vi "Lab Panel V4.85.vi"() -> ()   [LabVIEW 2013] (continued)
                    n1929 = Unbundle By Name(w3325) -> ("1  (A) cal"=w3318:dbl, "1 (V) cal"=w3317:dbl, "1 (PF) cal"=w3316:dbl, "2 (A) cal"=w3315:dbl, "2 (V) cal"=w3314:dbl, "2 (PF) cal"=w3313:dbl)  [unwired: 4 out]
                    n1930 = Multiply(x=w3324, y=w3318) -> (x*y=w3311:dbl)
                    n1931 = Multiply(x=w3323, y=w3317) -> (x*y=w3310:dbl)
                    n1932 = Multiply(x=w3322, y=w3316) -> (x*y=w3309:dbl)
                    n1933 = Multiply(x=w3321, y=w3315) -> (x*y=w3307:dbl)
                    n1934 = Multiply(x=w3320, y=w3314) -> (x*y=w3306:dbl)
                    n1935 = Multiply(x=w3319, y=w3313) -> (x*y=w3305:dbl)
                    n1936 = local read "SIG LAB04-1"() -> (w3312:T2)
                    n1937 = local read "SIG LAB04-2"() -> (w3308:T2)
                    n1938 = Bundle By Name(cluster=w3312, "AMPS"=w3311, "VOLTS"=w3310, "PF"=w3309) -> (w3301:T2)
                    n1939 = Bundle By Name(cluster=w3308, "AMPS"=w3307, "VOLTS"=w3306, "PF"=w3305) -> (w3300:T2)
                    n1940 = global write "Global display 1.vi" "SIG LAB04-2"(w3300) -> ()
                    n1941 = global write "Global display 1.vi" "SIG LAB04-1"(w3301) -> ()
                    n1942 = local write "SIG LAB04-2"(w3300) -> ()
                    n1943 = local write "SIG LAB04-1"(w3301) -> ()
                  }
                  frame #5 {
                    n1944 = Unbundle By Name(w3333) -> ("LAB05-1 (A)"=w3352:dbl, "LAB05-1 (V)"=w3332:dbl, "LAB05-1 (PF)"=w3351:dbl, "LAB05-2 (A)"=w3350:dbl, "LAB05-2 (V)"=w3349:dbl, "LAB05-2 (PF)"=w3348:dbl)
                    n1945 = case shown="False" w3331 {
                      tunnel: [w3354 w3355] -> w3353
                      tunnel: w3330 -> [_ w3355]
                      frame False {
                        n1946 = local read "CAL LAB05"() -> (w3354:T12)
                      }
                      frame True {
                      }
                    }
                    n1947 = Unbundle By Name(w3353) -> ("1  (A) cal"=w3347:dbl, "1 (V) cal"=w3346:dbl, "1 (PF) cal"=w3345:dbl, "2 (A) cal"=w3344:dbl, "2 (V) cal"=w3343:dbl, "2 (PF) cal"=w3342:dbl)  [unwired: 4 out]
                    n1948 = Multiply(x=w3352, y=w3347) -> (x*y=w3340:dbl)
                    n1949 = Multiply(x=w3332, y=w3346) -> (x*y=w3339:dbl)
                    n1950 = Multiply(x=w3351, y=w3345) -> (x*y=w3338:dbl)
                    n1951 = Multiply(x=w3350, y=w3344) -> (x*y=w3336:dbl)
                    n1952 = Multiply(x=w3349, y=w3343) -> (x*y=w3335:dbl)
                    n1953 = Multiply(x=w3348, y=w3342) -> (x*y=w3334:dbl)
                    n1954 = local read "SIG LAB05-1"() -> (w3341:T2)
                    n1955 = local read "SIG LAB05-2"() -> (w3337:T2)
                    n1956 = Bundle By Name(cluster=w3341, "AMPS"=w3340, "VOLTS"=w3339, "PF"=w3338) -> (w3329:T2)
                    n1957 = Bundle By Name(cluster=w3337, "AMPS"=w3336, "VOLTS"=w3335, "PF"=w3334) -> (w3328:T2)
                    n1958 = global write "Global display 1.vi" "SIG LAB05-1"(w3329) -> ()
                    n1959 = global write "Global display 1.vi" "SIG LAB05-2"(w3328) -> ()
                    n1960 = local write "SIG LAB05-2"(w3328) -> ()
                    n1961 = local write "SIG LAB05-1"(w3329) -> ()
                  }
                }
              }
            }
          }
          frame #12 {
            # "save test data to file"
            n1962 = Get Date/Time In Seconds() -> (seconds since 1Jan1904=w3356:timestamp)
            "File Time Stamp" <- w3356
            n1963 = local read "on loops"() -> (w3375:dbl)
            n1964 = local read "jig cycle"() -> (w3372:dbl)
            n1965 = Format Date/Time String(time format string (%c)="%H:%M%:%S", seconds (now)=w3356) -> (date/time string=w3360:string)  [unwired: 1 in]
            n1966 = Add(x=w3375, y=2) -> (x+y=w3373:dbl)
            n1967 = Build Array(w3360) -> (w3359:string[])
            n1968 = Equal?(x=w3372, y=1) -> (x = y?=w3358:bool)
            n1969 = Equal?(x=w3372, y=w3373) -> (x = y?=w3357:bool)
            n1970 = stacked-sequence {
              tunnel: w3371 -> [w3381 _ _ _ _ _ _ _ _ _]
              tunnel: w3370 -> [_ w3457 _ _ _ _ _ _ _ _]
              tunnel: w3369 -> [_ _ w3537 _ _ _ _ _ _ _]
              tunnel: w3368 -> [_ _ _ w3617 _ _ _ _ _ _]
              tunnel: w3367 -> [_ _ _ _ w3697 _ _ _ _ _]
              tunnel: w3366 -> [_ _ _ _ _ w3777 _ _ _ _]
              tunnel: w3365 -> [_ _ _ _ _ _ w3857 _ _ _]
              tunnel: w3364 -> [_ _ _ _ _ _ _ w3937 _ _]
              tunnel: w3363 -> [_ _ _ _ _ _ _ _ w4017 _]
              tunnel: w3362 -> [_ _ _ _ _ _ _ _ _ w4097]
              tunnel: w3359 -> [w3380 w3461 w3541 w3621 w3701 w3781 w3861 w3941 w4021 w4101]
              tunnel: w3358 -> [w3379 w3460 w3540 w3620 w3700 w3780 w3860 w3940 w4020 w4100]
              tunnel: w3357 -> [w3378 w3459 w3539 w3619 w3699 w3779 w3859 w3939 w4019 w4099]
              tunnel: w3356 -> [w3377 w3458 w3538 w3618 w3698 w3778 w3858 w3938 w4018 w4098]
              frame #0 {
                n1971 = case shown="True" w3381 {
                  tunnel: w3380 -> [_ w3386]
                  tunnel: w3379 -> [_ w3385]
                  tunnel: w3378 -> [_ w3383]
                  tunnel: w3377 -> [_ w3382]
                  frame False {
                  }
                  frame True {
                    n1972 = local read "DISP LAB01-1"() -> (w3387:T4)
                    n1973 = local read "SIG LAB01-1"() -> (w3388:T2)
                    n1974 = local read "ON L01-1"() -> (w3384:cluster{"amps":dbl, "volts":dbl, "pf":dbl})
                    n1975 = Unbundle(w3388) -> ("AMPS"=w3394:dbl, "VOLTS"=w3392:dbl, "PF"=w3391:dbl, "Tmp Live"=w3390:dbl, "Tmp Neut"=w3393:dbl)
                    n1976 = Unbundle(w3387) -> ("CYCLE"=w3389:dbl)  [unwired: 2 out]
                    n1977 = stacked-sequence {
                      tunnel: w3394 -> [w3398 w3417]
                      tunnel: w3393 -> [_ w3416]
                      tunnel: w3392 -> [w3397 w3415]
                      tunnel: w3391 -> [w3396 w3414]
                      tunnel: w3390 -> [_ w3413]
                      tunnel: w3389 -> [_ w3412]
                      tunnel: w3386 -> [_ w3411]
                      tunnel: w3385 -> [w3399 _]
                      tunnel: w3384 -> [w3395 w3409]
                      tunnel: w3383 -> [_ w3410]
                      tunnel: w3382 -> [_ w3405]
                      frame #0 {
                        n1978 = case shown="True" w3399 {
                          tunnel: w3398 -> [_ w3404]
                          tunnel: w3397 -> [_ w3403]
                          tunnel: w3396 -> [_ w3402]
                          tunnel: w3395 -> [_ w3400]
                          frame False {
                          }
                          frame True {
                            n1979 = Bundle(cluster=w3400, "amps"=w3404, "volts"=w3403, "pf"=w3402) -> (w3401:cluster{"amps":dbl, "volts":dbl, "pf":dbl})
                            n1980 = local write "ON L01-1"(w3401) -> ()
                          }
                        }
                      }
                      frame #1 {
                        n1981 = Unbundle(w3409) -> ("amps"=w3408:dbl, "volts"=w3407:dbl, "pf"=w3406:dbl)
                        n1982 = case shown="True" w3410 {
                          tunnel: w3417 -> [_ w3418]
                          tunnel: w3416 -> [_ w3456]
                          tunnel: w3415 -> [_ _]
                          tunnel: w3414 -> [_ _]
                          tunnel: w3413 -> [_ w3455]
                          tunnel: w3412 -> [_ w3454]
                          tunnel: w3411 -> [_ w3422]
                          tunnel: w3408 -> [_ w3419]
                          tunnel: w3407 -> [_ w3451]
                          tunnel: w3406 -> [_ w3450]
                          tunnel: w3405 -> [_ w3420]
                          frame False {
                          }
                          frame True {
                            n1983 = local read "TDMS LAB01-1"() -> (w3453:refnum<k34>)
                            n1984 = Build Array(w3451) -> (w3447:dbl[])
                            n1985 = Build Array(w3450) -> (w3446:dbl[])
                            n1986 = Build Array(w3455) -> (w3445:dbl[])
                            n1987 = Build Array(w3456) -> (w3444:dbl[])
                            n1988 = Build Array(w3419) -> (w3449:dbl[])
                            n1989 = Build Array(w3418) -> (w3448:dbl[])
                            n1990 = Build Array(w3454) -> (w3443:dbl[])
                            n1991 = Build Array("AMPS ON", "AMPS OFF", "VOLTS", "PF", "TEMP Live", "TEMP Neut", "CYCLE") -> (w3427:string[])
                            n1992 = Bundle By Name("Y"=w3449, "t0"=w3420) -> (w3442:waveform(dbl))  [unwired: 1 in]
                            n1993 = Bundle By Name("Y"=w3448, "t0"=w3420) -> (w3441:waveform(dbl))  [unwired: 1 in]
                            n1994 = Bundle By Name("Y"=w3447, "t0"=w3420) -> (w3440:waveform(dbl))  [unwired: 1 in]
                            n1995 = Bundle By Name("Y"=w3446, "t0"=w3420) -> (w3439:waveform(dbl))  [unwired: 1 in]
                            n1996 = Bundle By Name("Y"=w3445, "t0"=w3420) -> (w3438:waveform(dbl))  [unwired: 1 in]
                            n1997 = Bundle By Name("Y"=w3444, "t0"=w3420) -> (w3437:waveform(dbl))  [unwired: 1 in]
                            n1998 = Bundle By Name("Y"=w3443, "t0"=w3420) -> (w3436:waveform(dbl))  [unwired: 1 in]
                            n1999 = Build Array(w3442, w3441, w3440, w3439, w3438, w3437, w3436) -> (w3435:waveform(dbl)[])
                            n2000 = TDMS Write(0:w3453, 5:"TEST VALUES", 7:w3427, 9:w3435) -> (4:w3426:refnum<k34>, 6:w3425:string, 15:w3424:errorcluster)  [unwired: 2 in, 1 out]
                            n2001 = TDMS Write(0:w3426, 5:w3425, 7:"TIME", 9:w3422, 11:w3424) -> (15:w3421:errorcluster)  [unwired: 1 in, 3 out]
                            n2002 = local write "data file error"(w3421) -> ()
                          }
                        }
                      }
                    }
                  }
                }
              }
              frame #1 {
                n2003 = case shown="True" w3457 {
                  tunnel: w3461 -> [_ w3466]
                  tunnel: w3460 -> [_ w3465]
                  tunnel: w3459 -> [_ w3463]
                  tunnel: w3458 -> [_ w3462]
                  frame False {
                  }
                  frame True {
                    n2004 = local read "DISP LAB01-2"() -> (w3467:T4)
                    n2005 = local read "SIG LAB01-2"() -> (w3468:T2)
                    n2006 = local read "ON L01-2"() -> (w3464:cluster{"amps":dbl, "volts":dbl, "pf":dbl})
                    n2007 = Unbundle(w3468) -> ("AMPS"=w3474:dbl, "VOLTS"=w3472:dbl, "PF"=w3471:dbl, "Tmp Live"=w3470:dbl, "Tmp Neut"=w3473:dbl)
                    n2008 = Unbundle(w3467) -> ("CYCLE"=w3469:dbl)  [unwired: 2 out]
                    n2009 = stacked-sequence {
                      tunnel: w3474 -> [w3478 w3497]
                      tunnel: w3473 -> [_ w3496]
                      tunnel: w3472 -> [w3477 w3495]
                      tunnel: w3471 -> [w3476 w3494]
                      tunnel: w3470 -> [_ w3493]
                      tunnel: w3469 -> [_ w3492]
                      tunnel: w3466 -> [_ w3491]
                      tunnel: w3465 -> [w3479 _]
                      tunnel: w3464 -> [w3475 w3489]
                      tunnel: w3463 -> [_ w3490]
                      tunnel: w3462 -> [_ w3485]
                      frame #0 {
                        n2010 = case shown="True" w3479 {
                          tunnel: w3478 -> [_ w3484]
                          tunnel: w3477 -> [_ w3483]
                          tunnel: w3476 -> [_ w3482]
                          tunnel: w3475 -> [_ w3480]
                          frame False {
                          }
                          frame True {
                            n2011 = Bundle(cluster=w3480, "amps"=w3484, "volts"=w3483, "pf"=w3482) -> (w3481:cluster{"amps":dbl, "volts":dbl, "pf":dbl})
                            n2012 = local write "ON L01-2"(w3481) -> ()
                          }
                        }
                      }
                      frame #1 {
                        n2013 = Unbundle(w3489) -> ("amps"=w3488:dbl, "volts"=w3487:dbl, "pf"=w3486:dbl)
                        n2014 = case shown="True" w3490 {
                          tunnel: w3497 -> [_ w3529]
                          tunnel: w3496 -> [_ w3536]
                          tunnel: w3495 -> [_ _]
                          tunnel: w3494 -> [_ _]
                          tunnel: w3493 -> [_ w3535]
                          tunnel: w3492 -> [_ w3534]
                          tunnel: w3491 -> [_ w3499]
                          tunnel: w3488 -> [_ w3531]
                          tunnel: w3487 -> [_ w3530]
                          tunnel: w3486 -> [_ w3528]
                          tunnel: w3485 -> [_ w3520]
                          frame False {
                          }
                          frame True {
                            n2015 = local read "TDMS LAB01-2"() -> (w3533:refnum<k34>)
                            n2016 = Build Array(w3530) -> (w3525:dbl[])
                            n2017 = Build Array(w3528) -> (w3524:dbl[])
                            n2018 = Build Array(w3535) -> (w3523:dbl[])
                            n2019 = Build Array(w3536) -> (w3522:dbl[])
                            n2020 = Build Array(w3531) -> (w3527:dbl[])
                            n2021 = Build Array(w3529) -> (w3526:dbl[])
                            n2022 = Build Array(w3534) -> (w3521:dbl[])
                            n2023 = Build Array("AMPS ON", "AMPS OFF", "VOLTS", "PF", "TEMP Live", "TEMP Neut", "CYCLE") -> (w3504:string[])
                            n2024 = Bundle By Name("Y"=w3527, "t0"=w3520) -> (w3519:waveform(dbl))  [unwired: 1 in]
                            n2025 = Bundle By Name("Y"=w3526, "t0"=w3520) -> (w3518:waveform(dbl))  [unwired: 1 in]
                            n2026 = Bundle By Name("Y"=w3525, "t0"=w3520) -> (w3517:waveform(dbl))  [unwired: 1 in]
                            n2027 = Bundle By Name("Y"=w3524, "t0"=w3520) -> (w3516:waveform(dbl))  [unwired: 1 in]
                            n2028 = Bundle By Name("Y"=w3523, "t0"=w3520) -> (w3515:waveform(dbl))  [unwired: 1 in]
                            n2029 = Bundle By Name("Y"=w3522, "t0"=w3520) -> (w3514:waveform(dbl))  [unwired: 1 in]
                            n2030 = Bundle By Name("Y"=w3521, "t0"=w3520) -> (w3513:waveform(dbl))  [unwired: 1 in]
                            n2031 = Build Array(w3519, w3518, w3517, w3516, w3515, w3514, w3513) -> (w3512:waveform(dbl)[])
                            n2032 = TDMS Write(0:w3533, 5:"TEST VALUES", 7:w3504, 9:w3512) -> (4:w3503:refnum<k34>, 6:w3502:string, 15:w3501:errorcluster)  [unwired: 2 in, 1 out]
                            n2033 = TDMS Write(0:w3503, 5:w3502, 7:"TIME", 9:w3499, 11:w3501) -> (15:w3498:errorcluster)  [unwired: 1 in, 3 out]
                            n2034 = local write "data file error"(w3498) -> ()
                          }
                        }
                      }
                    }
                  }
                }
              }
              frame #2 {
                n2035 = case shown="True" w3537 {
                  tunnel: w3541 -> [_ w3546]
                  tunnel: w3540 -> [_ w3545]
                  tunnel: w3539 -> [_ w3543]
                  tunnel: w3538 -> [_ w3542]
                  frame False {
                  }
                  frame True {
                    n2036 = local read "DISP LAB02-1"() -> (w3547:T4)
                    n2037 = local read "SIG LAB02-1"() -> (w3548:T2)
                    n2038 = local read "ON L02-1"() -> (w3544:cluster{"amps":dbl, "volts":dbl, "pf":dbl})
                    n2039 = Unbundle(w3548) -> ("AMPS"=w3554:dbl, "VOLTS"=w3552:dbl, "PF"=w3551:dbl, "Tmp Live"=w3550:dbl, "Tmp Neut"=w3553:dbl)
                    n2040 = Unbundle(w3547) -> ("CYCLE"=w3549:dbl)  [unwired: 2 out]
                    n2041 = stacked-sequence {
                      tunnel: w3554 -> [w3558 w3577]
                      tunnel: w3553 -> [_ w3576]
                      tunnel: w3552 -> [w3557 w3575]
                      tunnel: w3551 -> [w3556 w3574]
                      tunnel: w3550 -> [_ w3573]
                      tunnel: w3549 -> [_ w3572]
                      tunnel: w3546 -> [_ w3571]
                      tunnel: w3545 -> [w3559 _]
                      tunnel: w3544 -> [w3555 w3569]
                      tunnel: w3543 -> [_ w3570]
                      tunnel: w3542 -> [_ w3565]
                      frame #0 {
                        n2042 = case shown="True" w3559 {
                          tunnel: w3558 -> [_ w3564]
                          tunnel: w3557 -> [_ w3563]
                          tunnel: w3556 -> [_ w3562]
                          tunnel: w3555 -> [_ w3560]
                          frame False {
                          }
                          frame True {
                            n2043 = Bundle(cluster=w3560, "amps"=w3564, "volts"=w3563, "pf"=w3562) -> (w3561:cluster{"amps":dbl, "volts":dbl, "pf":dbl})
                            n2044 = local write "ON L02-1"(w3561) -> ()
                          }
                        }
                      }
                      frame #1 {
                        n2045 = Unbundle(w3569) -> ("amps"=w3568:dbl, "volts"=w3567:dbl, "pf"=w3566:dbl)
                        n2046 = case shown="True" w3570 {
                          tunnel: w3577 -> [_ w3609]
                          tunnel: w3576 -> [_ w3616]
                          tunnel: w3575 -> [_ _]
                          tunnel: w3574 -> [_ _]
                          tunnel: w3573 -> [_ w3615]
                          tunnel: w3572 -> [_ w3614]
                          tunnel: w3571 -> [_ w3579]
                          tunnel: w3568 -> [_ w3611]
                          tunnel: w3567 -> [_ w3610]
                          tunnel: w3566 -> [_ w3608]
                          tunnel: w3565 -> [_ w3600]
                          frame False {
                          }
                          frame True {
                            n2047 = local read "TDMS LAB02-1"() -> (w3613:refnum<k34>)
                            n2048 = Build Array(w3610) -> (w3605:dbl[])
                            n2049 = Build Array(w3608) -> (w3604:dbl[])
                            n2050 = Build Array(w3615) -> (w3603:dbl[])
                            n2051 = Build Array(w3616) -> (w3602:dbl[])
                            n2052 = Build Array(w3611) -> (w3607:dbl[])
                            n2053 = Build Array(w3609) -> (w3606:dbl[])
                            n2054 = Build Array(w3614) -> (w3601:dbl[])
                            n2055 = Build Array("AMPS ON", "AMPS OFF", "VOLTS", "PF", "TEMP Live", "TEMP Neut", "CYCLE") -> (w3584:string[])
                            n2056 = Bundle By Name("Y"=w3607, "t0"=w3600) -> (w3599:waveform(dbl))  [unwired: 1 in]
                            n2057 = Bundle By Name("Y"=w3606, "t0"=w3600) -> (w3598:waveform(dbl))  [unwired: 1 in]
                            n2058 = Bundle By Name("Y"=w3605, "t0"=w3600) -> (w3597:waveform(dbl))  [unwired: 1 in]
                            n2059 = Bundle By Name("Y"=w3604, "t0"=w3600) -> (w3596:waveform(dbl))  [unwired: 1 in]
                            n2060 = Bundle By Name("Y"=w3603, "t0"=w3600) -> (w3595:waveform(dbl))  [unwired: 1 in]
                            n2061 = Bundle By Name("Y"=w3602, "t0"=w3600) -> (w3594:waveform(dbl))  [unwired: 1 in]
                            n2062 = Bundle By Name("Y"=w3601, "t0"=w3600) -> (w3593:waveform(dbl))  [unwired: 1 in]
                            n2063 = Build Array(w3599, w3598, w3597, w3596, w3595, w3594, w3593) -> (w3592:waveform(dbl)[])
                            n2064 = TDMS Write(0:w3613, 5:"TEST VALUES", 7:w3584, 9:w3592) -> (4:w3583:refnum<k34>, 6:w3582:string, 15:w3581:errorcluster)  [unwired: 2 in, 1 out]
                            n2065 = TDMS Write(0:w3583, 5:w3582, 7:"TIME", 9:w3579, 11:w3581) -> (15:w3578:errorcluster)  [unwired: 1 in, 3 out]
                            n2066 = local write "data file error"(w3578) -> ()
                          }
                        }
                      }
                    }
                  }
                }
              }
              frame #3 {
                n2067 = case shown="True" w3617 {
                  tunnel: w3621 -> [_ w3626]
                  tunnel: w3620 -> [_ w3625]
                  tunnel: w3619 -> [_ w3623]
                  tunnel: w3618 -> [_ w3622]
                  frame False {
                  }
                  frame True {
                    n2068 = local read "DISP LAB02-2"() -> (w3627:T4)
                    n2069 = local read "SIG LAB02-2"() -> (w3628:T2)
                    n2070 = local read "ON L02-2"() -> (w3624:cluster{"amps":dbl, "volts":dbl, "pf":dbl})
                    n2071 = Unbundle(w3628) -> ("AMPS"=w3634:dbl, "VOLTS"=w3632:dbl, "PF"=w3631:dbl, "Tmp Live"=w3630:dbl, "Tmp Neut"=w3633:dbl)
                    n2072 = Unbundle(w3627) -> ("CYCLE"=w3629:dbl)  [unwired: 2 out]
                    n2073 = stacked-sequence {
                      tunnel: w3634 -> [w3638 w3657]
                      tunnel: w3633 -> [_ w3656]
                      tunnel: w3632 -> [w3637 w3655]
                      tunnel: w3631 -> [w3636 w3654]
                      tunnel: w3630 -> [_ w3653]
                      tunnel: w3629 -> [_ w3652]
                      tunnel: w3626 -> [_ w3651]
                      tunnel: w3625 -> [w3639 _]
                      tunnel: w3624 -> [w3635 w3649]
                      tunnel: w3623 -> [_ w3650]
                      tunnel: w3622 -> [_ w3645]
                      frame #0 {
                        n2074 = case shown="True" w3639 {
                          tunnel: w3638 -> [_ w3644]
                          tunnel: w3637 -> [_ w3643]
                          tunnel: w3636 -> [_ w3642]
                          tunnel: w3635 -> [_ w3640]
                          frame False {
                          }
                          frame True {
                            n2075 = Bundle(cluster=w3640, "amps"=w3644, "volts"=w3643, "pf"=w3642) -> (w3641:cluster{"amps":dbl, "volts":dbl, "pf":dbl})
                            n2076 = local write "ON L02-2"(w3641) -> ()
                          }
                        }
                      }
                      frame #1 {
                        n2077 = Unbundle(w3649) -> ("amps"=w3648:dbl, "volts"=w3647:dbl, "pf"=w3646:dbl)
                        n2078 = case shown="True" w3650 {
                          tunnel: w3657 -> [_ w3689]
                          tunnel: w3656 -> [_ w3696]
                          tunnel: w3655 -> [_ _]
                          tunnel: w3654 -> [_ _]
                          tunnel: w3653 -> [_ w3695]
                          tunnel: w3652 -> [_ w3694]
                          tunnel: w3651 -> [_ w3659]
                          tunnel: w3648 -> [_ w3691]
                          tunnel: w3647 -> [_ w3690]
                          tunnel: w3646 -> [_ w3688]
                          tunnel: w3645 -> [_ w3680]
                          frame False {
                          }
                          frame True {
                            n2079 = local read "TDMS LAB02-2"() -> (w3693:refnum<k34>)
                            n2080 = Build Array(w3690) -> (w3685:dbl[])
                            n2081 = Build Array(w3688) -> (w3684:dbl[])
                            n2082 = Build Array(w3695) -> (w3683:dbl[])
                            n2083 = Build Array(w3696) -> (w3682:dbl[])
                            n2084 = Build Array(w3691) -> (w3687:dbl[])
                            n2085 = Build Array(w3689) -> (w3686:dbl[])
                            n2086 = Build Array(w3694) -> (w3681:dbl[])
                            n2087 = Build Array("AMPS ON", "AMPS OFF", "VOLTS", "PF", "TEMP Live", "TEMP Neut", "CYCLE") -> (w3664:string[])
                            n2088 = Bundle By Name("Y"=w3687, "t0"=w3680) -> (w3679:waveform(dbl))  [unwired: 1 in]
                            n2089 = Bundle By Name("Y"=w3686, "t0"=w3680) -> (w3678:waveform(dbl))  [unwired: 1 in]
                            n2090 = Bundle By Name("Y"=w3685, "t0"=w3680) -> (w3677:waveform(dbl))  [unwired: 1 in]
                            n2091 = Bundle By Name("Y"=w3684, "t0"=w3680) -> (w3676:waveform(dbl))  [unwired: 1 in]
                            n2092 = Bundle By Name("Y"=w3683, "t0"=w3680) -> (w3675:waveform(dbl))  [unwired: 1 in]
                            n2093 = Bundle By Name("Y"=w3682, "t0"=w3680) -> (w3674:waveform(dbl))  [unwired: 1 in]
                            n2094 = Bundle By Name("Y"=w3681, "t0"=w3680) -> (w3673:waveform(dbl))  [unwired: 1 in]
                            n2095 = Build Array(w3679, w3678, w3677, w3676, w3675, w3674, w3673) -> (w3672:waveform(dbl)[])
                            n2096 = TDMS Write(0:w3693, 5:"TEST VALUES", 7:w3664, 9:w3672) -> (4:w3663:refnum<k34>, 6:w3662:string, 15:w3661:errorcluster)  [unwired: 2 in, 1 out]
                            n2097 = TDMS Write(0:w3663, 5:w3662, 7:"TIME", 9:w3659, 11:w3661) -> (15:w3658:errorcluster)  [unwired: 1 in, 3 out]
                            n2098 = local write "data file error"(w3658) -> ()
                          }
                        }
                      }
                    }
                  }
                }
              }
              frame #4 {
                n2099 = case shown="True" w3697 {
                  tunnel: w3701 -> [_ w3706]
                  tunnel: w3700 -> [_ w3705]
                  tunnel: w3699 -> [_ w3703]
                  tunnel: w3698 -> [_ w3702]
                  frame False {
                  }
                  frame True {
                    n2100 = local read "DISP LAB03-1"() -> (w3707:T4)
                    n2101 = local read "SIG LAB03-1"() -> (w3708:T2)
                    n2102 = local read "ON L03-1"() -> (w3704:cluster{"amps":dbl, "volts":dbl, "pf":dbl})
                    n2103 = Unbundle(w3708) -> ("AMPS"=w3714:dbl, "VOLTS"=w3712:dbl, "PF"=w3711:dbl, "Tmp Live"=w3710:dbl, "Tmp Neut"=w3713:dbl)
                    n2104 = Unbundle(w3707) -> ("CYCLE"=w3709:dbl)  [unwired: 2 out]
                    n2105 = stacked-sequence {
                      tunnel: w3714 -> [w3718 w3737]
                      tunnel: w3713 -> [_ w3736]
                      tunnel: w3712 -> [w3717 w3735]
                      tunnel: w3711 -> [w3716 w3734]
                      tunnel: w3710 -> [_ w3733]
                      tunnel: w3709 -> [_ w3732]
                      tunnel: w3706 -> [_ w3731]
                      tunnel: w3705 -> [w3719 _]
                      tunnel: w3704 -> [w3715 w3729]
                      tunnel: w3703 -> [_ w3730]
                      tunnel: w3702 -> [_ w3725]
                      frame #0 {
                        n2106 = case shown="True" w3719 {
                          tunnel: w3718 -> [_ w3724]
                          tunnel: w3717 -> [_ w3723]
                          tunnel: w3716 -> [_ w3722]
                          tunnel: w3715 -> [_ w3720]
                          frame False {
                          }
                          frame True {
                            n2107 = Bundle(cluster=w3720, "amps"=w3724, "volts"=w3723, "pf"=w3722) -> (w3721:cluster{"amps":dbl, "volts":dbl, "pf":dbl})
                            n2108 = local write "ON L03-1"(w3721) -> ()
                          }
                        }
                      }
                      frame #1 {
                        n2109 = Unbundle(w3729) -> ("amps"=w3728:dbl, "volts"=w3727:dbl, "pf"=w3726:dbl)
                        n2110 = case shown="True" w3730 {
                          tunnel: w3737 -> [_ w3769]
                          tunnel: w3736 -> [_ w3776]
                          tunnel: w3735 -> [_ _]
                          tunnel: w3734 -> [_ _]
                          tunnel: w3733 -> [_ w3775]
                          tunnel: w3732 -> [_ w3774]
                          tunnel: w3731 -> [_ w3739]
                          tunnel: w3728 -> [_ w3771]
                          tunnel: w3727 -> [_ w3770]
                          tunnel: w3726 -> [_ w3768]
                          tunnel: w3725 -> [_ w3760]
                          frame False {
                          }
                          frame True {
                            n2111 = local read "TDMS LAB03-1"() -> (w3773:refnum<k34>)
                            n2112 = Build Array(w3770) -> (w3765:dbl[])
                            n2113 = Build Array(w3768) -> (w3764:dbl[])
                            n2114 = Build Array(w3775) -> (w3763:dbl[])
                            n2115 = Build Array(w3776) -> (w3762:dbl[])
                            n2116 = Build Array(w3771) -> (w3767:dbl[])
                            n2117 = Build Array(w3769) -> (w3766:dbl[])
                            n2118 = Build Array(w3774) -> (w3761:dbl[])
                            n2119 = Build Array("AMPS ON", "AMPS OFF", "VOLTS", "PF", "TEMP Live", "TEMP Neut", "CYCLE") -> (w3744:string[])
                            n2120 = Bundle By Name("Y"=w3767, "t0"=w3760) -> (w3759:waveform(dbl))  [unwired: 1 in]
                            n2121 = Bundle By Name("Y"=w3766, "t0"=w3760) -> (w3758:waveform(dbl))  [unwired: 1 in]
                            n2122 = Bundle By Name("Y"=w3765, "t0"=w3760) -> (w3757:waveform(dbl))  [unwired: 1 in]
                            n2123 = Bundle By Name("Y"=w3764, "t0"=w3760) -> (w3756:waveform(dbl))  [unwired: 1 in]
                            n2124 = Bundle By Name("Y"=w3763, "t0"=w3760) -> (w3755:waveform(dbl))  [unwired: 1 in]
                            n2125 = Bundle By Name("Y"=w3762, "t0"=w3760) -> (w3754:waveform(dbl))  [unwired: 1 in]
                            n2126 = Bundle By Name("Y"=w3761, "t0"=w3760) -> (w3753:waveform(dbl))  [unwired: 1 in]
                            n2127 = Build Array(w3759, w3758, w3757, w3756, w3755, w3754, w3753) -> (w3752:waveform(dbl)[])
                            n2128 = TDMS Write(0:w3773, 5:"TEST VALUES", 7:w3744, 9:w3752) -> (4:w3743:refnum<k34>, 6:w3742:string, 15:w3741:errorcluster)  [unwired: 2 in, 1 out]
                            n2129 = TDMS Write(0:w3743, 5:w3742, 7:"TIME", 9:w3739, 11:w3741) -> (15:w3738:errorcluster)  [unwired: 1 in, 3 out]
                            n2130 = local write "data file error"(w3738) -> ()
                          }
                        }
                      }
                    }
                  }
                }
              }
              frame #5 {
                n2131 = case shown="True" w3777 {
                  tunnel: w3781 -> [_ w3786]
                  tunnel: w3780 -> [_ w3785]
                  tunnel: w3779 -> [_ w3783]
                  tunnel: w3778 -> [_ w3782]
                  frame False {
                  }
                  frame True {
                    n2132 = local read "DISP LAB03-2"() -> (w3787:T4)
                    n2133 = local read "SIG LAB03-2"() -> (w3788:T2)
                    n2134 = local read "ON L03-2"() -> (w3784:cluster{"amps":dbl, "volts":dbl, "pf":dbl})
                    n2135 = Unbundle(w3788) -> ("AMPS"=w3794:dbl, "VOLTS"=w3792:dbl, "PF"=w3791:dbl, "Tmp Live"=w3790:dbl, "Tmp Neut"=w3793:dbl)
                    n2136 = Unbundle(w3787) -> ("CYCLE"=w3789:dbl)  [unwired: 2 out]
                    n2137 = stacked-sequence {
                      tunnel: w3794 -> [w3798 w3817]
                      tunnel: w3793 -> [_ w3816]
                      tunnel: w3792 -> [w3797 w3815]
                      tunnel: w3791 -> [w3796 w3814]
                      tunnel: w3790 -> [_ w3813]
                      tunnel: w3789 -> [_ w3812]
                      tunnel: w3786 -> [_ w3811]
                      tunnel: w3785 -> [w3799 _]
                      tunnel: w3784 -> [w3795 w3809]
                      tunnel: w3783 -> [_ w3810]
                      tunnel: w3782 -> [_ w3805]
                      frame #0 {
                        n2138 = case shown="True" w3799 {
                          tunnel: w3798 -> [_ w3804]
                          tunnel: w3797 -> [_ w3803]
                          tunnel: w3796 -> [_ w3802]
                          tunnel: w3795 -> [_ w3800]
                          frame False {
                          }
                          frame True {
                            n2139 = Bundle(cluster=w3800, "amps"=w3804, "volts"=w3803, "pf"=w3802) -> (w3801:cluster{"amps":dbl, "volts":dbl, "pf":dbl})
                            n2140 = local write "ON L03-2"(w3801) -> ()
                          }
                        }
                      }
                      frame #1 {
                        n2141 = Unbundle(w3809) -> ("amps"=w3808:dbl, "volts"=w3807:dbl, "pf"=w3806:dbl)
                        n2142 = case shown="True" w3810 {
                          tunnel: w3817 -> [_ w3849]
                          tunnel: w3816 -> [_ w3856]
                          tunnel: w3815 -> [_ _]
                          tunnel: w3814 -> [_ _]
                          tunnel: w3813 -> [_ w3855]
                          tunnel: w3812 -> [_ w3854]
                          tunnel: w3811 -> [_ w3819]
                          tunnel: w3808 -> [_ w3851]
                          tunnel: w3807 -> [_ w3850]
                          tunnel: w3806 -> [_ w3848]
                          tunnel: w3805 -> [_ w3840]
                          frame False {
                          }
                          frame True {
                            n2143 = local read "TDMS LAB03-2"() -> (w3853:refnum<k34>)
                            n2144 = Build Array(w3850) -> (w3845:dbl[])
                            n2145 = Build Array(w3848) -> (w3844:dbl[])
                            n2146 = Build Array(w3855) -> (w3843:dbl[])
                            n2147 = Build Array(w3856) -> (w3842:dbl[])
                            n2148 = Build Array(w3851) -> (w3847:dbl[])
                            n2149 = Build Array(w3849) -> (w3846:dbl[])
                            n2150 = Build Array(w3854) -> (w3841:dbl[])
                            n2151 = Build Array("AMPS ON", "AMPS OFF", "VOLTS", "PF", "TEMP Live", "TEMP Neut", "CYCLE") -> (w3824:string[])
                            n2152 = Bundle By Name("Y"=w3847, "t0"=w3840) -> (w3839:waveform(dbl))  [unwired: 1 in]
                            n2153 = Bundle By Name("Y"=w3846, "t0"=w3840) -> (w3838:waveform(dbl))  [unwired: 1 in]
                            n2154 = Bundle By Name("Y"=w3845, "t0"=w3840) -> (w3837:waveform(dbl))  [unwired: 1 in]
                            n2155 = Bundle By Name("Y"=w3844, "t0"=w3840) -> (w3836:waveform(dbl))  [unwired: 1 in]
                            n2156 = Bundle By Name("Y"=w3843, "t0"=w3840) -> (w3835:waveform(dbl))  [unwired: 1 in]
                            n2157 = Bundle By Name("Y"=w3842, "t0"=w3840) -> (w3834:waveform(dbl))  [unwired: 1 in]
                            n2158 = Bundle By Name("Y"=w3841, "t0"=w3840) -> (w3833:waveform(dbl))  [unwired: 1 in]
                            n2159 = Build Array(w3839, w3838, w3837, w3836, w3835, w3834, w3833) -> (w3832:waveform(dbl)[])
                            n2160 = TDMS Write(0:w3853, 5:"TEST VALUES", 7:w3824, 9:w3832) -> (4:w3823:refnum<k34>, 6:w3822:string, 15:w3821:errorcluster)  [unwired: 2 in, 1 out]
                            n2161 = TDMS Write(0:w3823, 5:w3822, 7:"TIME", 9:w3819, 11:w3821) -> (15:w3818:errorcluster)  [unwired: 1 in, 3 out]
                            n2162 = local write "data file error"(w3818) -> ()
                          }
                        }
                      }
                    }
                  }
                }
              }
              frame #6 {
                n2163 = case shown="True" w3857 {
                  tunnel: w3861 -> [_ w3866]
                  tunnel: w3860 -> [_ w3865]
                  tunnel: w3859 -> [_ w3863]
                  tunnel: w3858 -> [_ w3862]
                  frame False {
                  }
                  frame True {
                    n2164 = local read "DISP LAB04-1"() -> (w3867:T4)
                    n2165 = local read "SIG LAB04-1"() -> (w3868:T2)
                    n2166 = local read "ON L04-1"() -> (w3864:cluster{"amps":dbl, "volts":dbl, "pf":dbl})
                    n2167 = Unbundle(w3868) -> ("AMPS"=w3874:dbl, "VOLTS"=w3872:dbl, "PF"=w3871:dbl, "Tmp Live"=w3870:dbl, "Tmp Neut"=w3873:dbl)
                    n2168 = Unbundle(w3867) -> ("CYCLE"=w3869:dbl)  [unwired: 2 out]
                    n2169 = stacked-sequence {
                      tunnel: w3874 -> [w3878 w3897]
                      tunnel: w3873 -> [_ w3896]
                      tunnel: w3872 -> [w3877 w3895]
                      tunnel: w3871 -> [w3876 w3894]
                      tunnel: w3870 -> [_ w3893]
                      tunnel: w3869 -> [_ w3892]
                      tunnel: w3866 -> [_ w3891]
                      tunnel: w3865 -> [w3879 _]
                      tunnel: w3864 -> [w3875 w3889]
                      tunnel: w3863 -> [_ w3890]
                      tunnel: w3862 -> [_ w3885]
                      frame #0 {
                        n2170 = case shown="True" w3879 {
                          tunnel: w3878 -> [_ w3884]
                          tunnel: w3877 -> [_ w3883]
                          tunnel: w3876 -> [_ w3882]
                          tunnel: w3875 -> [_ w3880]
                          frame False {
                          }
                          frame True {
                            n2171 = Bundle(cluster=w3880, "amps"=w3884, "volts"=w3883, "pf"=w3882) -> (w3881:cluster{"amps":dbl, "volts":dbl, "pf":dbl})
                            n2172 = local write "ON L04-1"(w3881) -> ()
                          }
                        }
                      }
                      frame #1 {
                        n2173 = Unbundle(w3889) -> ("amps"=w3888:dbl, "volts"=w3887:dbl, "pf"=w3886:dbl)
                        n2174 = case shown="True" w3890 {
                          tunnel: w3897 -> [_ w3929]
                          tunnel: w3896 -> [_ w3936]
                          tunnel: w3895 -> [_ _]
                          tunnel: w3894 -> [_ _]
                          tunnel: w3893 -> [_ w3935]
                          tunnel: w3892 -> [_ w3934]
                          tunnel: w3891 -> [_ w3899]
                          tunnel: w3888 -> [_ w3931]
                          tunnel: w3887 -> [_ w3930]
                          tunnel: w3886 -> [_ w3928]
                          tunnel: w3885 -> [_ w3920]
                          frame False {
                          }
                          frame True {
                            n2175 = local read "TDMS LAB04-1"() -> (w3933:refnum<k34>)
                            n2176 = Build Array(w3930) -> (w3925:dbl[])
                            n2177 = Build Array(w3928) -> (w3924:dbl[])
                            n2178 = Build Array(w3935) -> (w3923:dbl[])
                            n2179 = Build Array(w3936) -> (w3922:dbl[])
                            n2180 = Build Array(w3931) -> (w3927:dbl[])
                            n2181 = Build Array(w3929) -> (w3926:dbl[])
                            n2182 = Build Array(w3934) -> (w3921:dbl[])
                            n2183 = Build Array("AMPS ON", "AMPS OFF", "VOLTS", "PF", "TEMP Live", "TEMP Neut", "CYCLE") -> (w3904:string[])
                            n2184 = Bundle By Name("Y"=w3927, "t0"=w3920) -> (w3919:waveform(dbl))  [unwired: 1 in]
                            n2185 = Bundle By Name("Y"=w3926, "t0"=w3920) -> (w3918:waveform(dbl))  [unwired: 1 in]
                            n2186 = Bundle By Name("Y"=w3925, "t0"=w3920) -> (w3917:waveform(dbl))  [unwired: 1 in]
                            n2187 = Bundle By Name("Y"=w3924, "t0"=w3920) -> (w3916:waveform(dbl))  [unwired: 1 in]
                            n2188 = Bundle By Name("Y"=w3923, "t0"=w3920) -> (w3915:waveform(dbl))  [unwired: 1 in]
                            n2189 = Bundle By Name("Y"=w3922, "t0"=w3920) -> (w3914:waveform(dbl))  [unwired: 1 in]
                            n2190 = Bundle By Name("Y"=w3921, "t0"=w3920) -> (w3913:waveform(dbl))  [unwired: 1 in]
                            n2191 = Build Array(w3919, w3918, w3917, w3916, w3915, w3914, w3913) -> (w3912:waveform(dbl)[])
                            n2192 = TDMS Write(0:w3933, 5:"TEST VALUES", 7:w3904, 9:w3912) -> (4:w3903:refnum<k34>, 6:w3902:string, 15:w3901:errorcluster)  [unwired: 2 in, 1 out]
                            n2193 = TDMS Write(0:w3903, 5:w3902, 7:"TIME", 9:w3899, 11:w3901) -> (15:w3898:errorcluster)  [unwired: 1 in, 3 out]
                            n2194 = local write "data file error"(w3898) -> ()
                          }
                        }
                      }
                    }
                  }
                }
              }
              frame #7 {
                n2195 = case shown="True" w3937 {
                  tunnel: w3941 -> [_ w3946]
                  tunnel: w3940 -> [_ w3945]
                  tunnel: w3939 -> [_ w3943]
                  tunnel: w3938 -> [_ w3942]
                  frame False {
                  }
                  frame True {
                    n2196 = local read "DISP LAB04-2"() -> (w3947:T4)
                    n2197 = local read "SIG LAB04-2"() -> (w3948:T2)
                    n2198 = local read "ON L04-2"() -> (w3944:cluster{"amps":dbl, "volts":dbl, "pf":dbl})
                    n2199 = Unbundle(w3948) -> ("AMPS"=w3954:dbl, "VOLTS"=w3952:dbl, "PF"=w3951:dbl, "Tmp Live"=w3950:dbl, "Tmp Neut"=w3953:dbl)
                    n2200 = Unbundle(w3947) -> ("CYCLE"=w3949:dbl)  [unwired: 2 out]
                    n2201 = stacked-sequence {
                      tunnel: w3954 -> [w3958 w3977]
                      tunnel: w3953 -> [_ w3976]
                      tunnel: w3952 -> [w3957 w3975]
                      tunnel: w3951 -> [w3956 w3974]
                      tunnel: w3950 -> [_ w3973]
                      tunnel: w3949 -> [_ w3972]
                      tunnel: w3946 -> [_ w3971]
                      tunnel: w3945 -> [w3959 _]
                      tunnel: w3944 -> [w3955 w3969]
                      tunnel: w3943 -> [_ w3970]
                      tunnel: w3942 -> [_ w3965]
                      frame #0 {
                        n2202 = case shown="True" w3959 {
                          tunnel: w3958 -> [_ w3964]
                          tunnel: w3957 -> [_ w3963]
                          tunnel: w3956 -> [_ w3962]
                          tunnel: w3955 -> [_ w3960]
                          frame False {
                          }
                          frame True {
                            n2203 = Bundle(cluster=w3960, "amps"=w3964, "volts"=w3963, "pf"=w3962) -> (w3961:cluster{"amps":dbl, "volts":dbl, "pf":dbl})
                            n2204 = local write "ON L04-2"(w3961) -> ()
                          }
                        }
                      }
                      frame #1 {
                        n2205 = Unbundle(w3969) -> ("amps"=w3968:dbl, "volts"=w3967:dbl, "pf"=w3966:dbl)
                        n2206 = case shown="True" w3970 {
                          tunnel: w3977 -> [_ w4009]
                          tunnel: w3976 -> [_ w4016]
                          tunnel: w3975 -> [_ _]
                          tunnel: w3974 -> [_ _]
                          tunnel: w3973 -> [_ w4015]
                          tunnel: w3972 -> [_ w4014]
                          tunnel: w3971 -> [_ w3979]
                          tunnel: w3968 -> [_ w4011]
                          tunnel: w3967 -> [_ w4010]
                          tunnel: w3966 -> [_ w4008]
                          tunnel: w3965 -> [_ w4000]
                          frame False {
                          }
                          frame True {
                            n2207 = local read "TDMS LAB04-2"() -> (w4013:refnum<k34>)
                            n2208 = Build Array(w4010) -> (w4005:dbl[])
                            n2209 = Build Array(w4008) -> (w4004:dbl[])
                            n2210 = Build Array(w4015) -> (w4003:dbl[])
                            n2211 = Build Array(w4016) -> (w4002:dbl[])
                            n2212 = Build Array(w4011) -> (w4007:dbl[])
                            n2213 = Build Array(w4009) -> (w4006:dbl[])
                            n2214 = Build Array(w4014) -> (w4001:dbl[])
                            n2215 = Build Array("AMPS ON", "AMPS OFF", "VOLTS", "PF", "TEMP Live", "TEMP Neut", "CYCLE") -> (w3984:string[])
                            n2216 = Bundle By Name("Y"=w4007, "t0"=w4000) -> (w3999:waveform(dbl))  [unwired: 1 in]
                            n2217 = Bundle By Name("Y"=w4006, "t0"=w4000) -> (w3998:waveform(dbl))  [unwired: 1 in]
                            n2218 = Bundle By Name("Y"=w4005, "t0"=w4000) -> (w3997:waveform(dbl))  [unwired: 1 in]
                            n2219 = Bundle By Name("Y"=w4004, "t0"=w4000) -> (w3996:waveform(dbl))  [unwired: 1 in]
                            n2220 = Bundle By Name("Y"=w4003, "t0"=w4000) -> (w3995:waveform(dbl))  [unwired: 1 in]
                            n2221 = Bundle By Name("Y"=w4002, "t0"=w4000) -> (w3994:waveform(dbl))  [unwired: 1 in]
                            n2222 = Bundle By Name("Y"=w4001, "t0"=w4000) -> (w3993:waveform(dbl))  [unwired: 1 in]
                            n2223 = Build Array(w3999, w3998, w3997, w3996, w3995, w3994, w3993) -> (w3992:waveform(dbl)[])
                            n2224 = TDMS Write(0:w4013, 5:"TEST VALUES", 7:w3984, 9:w3992) -> (4:w3983:refnum<k34>, 6:w3982:string, 15:w3981:errorcluster)  [unwired: 2 in, 1 out]
                            n2225 = TDMS Write(0:w3983, 5:w3982, 7:"TIME", 9:w3979, 11:w3981) -> (15:w3978:errorcluster)  [unwired: 1 in, 3 out]
                            n2226 = local write "data file error"(w3978) -> ()
                          }
                        }
                      }
                    }
                  }
                }
              }
              frame #8 {
                n2227 = case shown="True" w4017 {
                  tunnel: w4021 -> [_ w4026]
                  tunnel: w4020 -> [_ w4025]
                  tunnel: w4019 -> [_ w4023]
                  tunnel: w4018 -> [_ w4022]
                  frame False {
                  }
                  frame True {
                    n2228 = local read "DISP LAB05-1"() -> (w4027:T4)
                    n2229 = local read "SIG LAB05-1"() -> (w4028:T2)
                    n2230 = local read "ON L05-1"() -> (w4024:cluster{"amps":dbl, "volts":dbl, "pf":dbl})
                    n2231 = Unbundle(w4028) -> ("AMPS"=w4034:dbl, "VOLTS"=w4032:dbl, "PF"=w4031:dbl, "Tmp Live"=w4030:dbl, "Tmp Neut"=w4033:dbl)
                    n2232 = Unbundle(w4027) -> ("CYCLE"=w4029:dbl)  [unwired: 2 out]
                    n2233 = stacked-sequence {
                      tunnel: w4034 -> [w4038 w4057]
                      tunnel: w4033 -> [_ w4056]
                      tunnel: w4032 -> [w4037 w4055]
                      tunnel: w4031 -> [w4036 w4054]
                      tunnel: w4030 -> [_ w4053]
                      tunnel: w4029 -> [_ w4052]
                      tunnel: w4026 -> [_ w4051]
                      tunnel: w4025 -> [w4039 _]
                      tunnel: w4024 -> [w4035 w4049]
                      tunnel: w4023 -> [_ w4050]
                      tunnel: w4022 -> [_ w4045]
                      frame #0 {
                        n2234 = case shown="True" w4039 {
                          tunnel: w4038 -> [_ w4044]
                          tunnel: w4037 -> [_ w4043]
                          tunnel: w4036 -> [_ w4042]
                          tunnel: w4035 -> [_ w4040]
                          frame False {
                          }
                          frame True {
